vi "Cleanup.vi"(8 "error in (no error)":errorcluster, 11 "Entity Manager in":refnum<class "Entity Manager.lvclass">) -> (0 "error out":errorcluster)   [LabVIEW 2020, in "Conditum.lvlib" / "Entity Manager.lvclass"]
uses:
  Entity Manager.lvclass
  Entity Manager.lvclass/Entity Manager.ctl
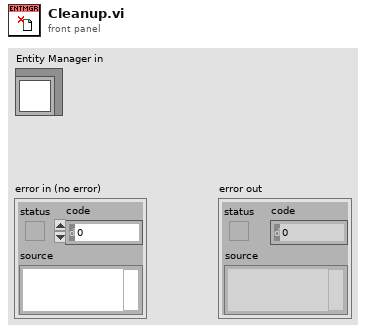
[diagram p1: front panel]
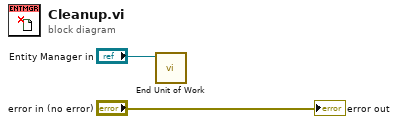
[diagram p0: block diagram]
diagram:
  n1 = call "End Unit of Work.vi"("Entity Manager in"="Entity Manager in") -> ()  [unwired: 9 in, 2 out]
  "error out" <- "error in (no error)"
